vi "Downloader.vi"(4 "port":u16=9090, 6 "address":string="192.168.1.7", 7 "Message Box":refnum<vi>, 8 "error in":errorcluster, 11 "source":path=path "") -> (0 "error out":errorcluster, 3 "Downloader out":refnum<class "Downloader.lvclass">)   [LabVIEW 2014, in "Raspberry Pi Compatible Compiler for LabVIEW.lvlib" / "Downloader.lvclass"]
uses:
  Downloader.lvclass
  Downloader.lvclass/Downloader.ctl
  MessageBox/MessageBox.lvclass
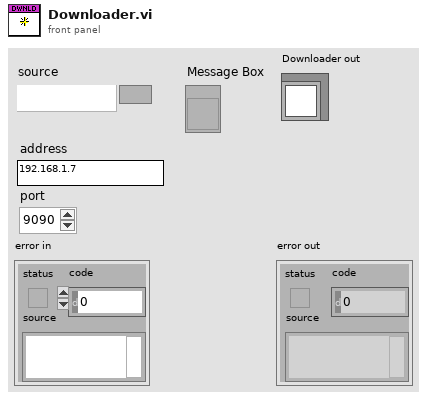
[diagram p1: front panel]
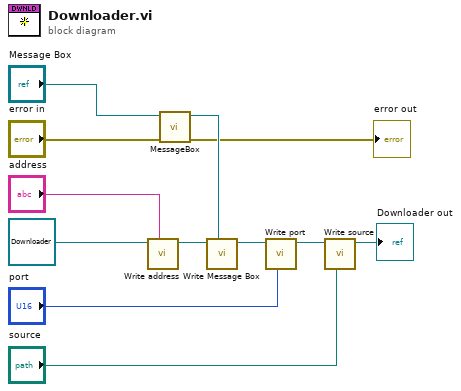
[diagram p0: block diagram]
diagram:
  n1 = call "Write address.vi"("address"="address", "Downloader in"=refnum<class "Downloader.lvclass"> refnum) -> ("Downloader out"=w12:refnum<class "Downloader.lvclass">)  [unwired: 7 in]
  n2 = call "MessageBox.vi"("error in"="error in", "Message Box"="Message Box") -> ("error out"=→"error out":errorcluster, "MessageBox out"=w3:refnum<class "MessageBox.lvclass">)  [unwired: 8 in]
  n3 = call "Write Message Box.vi"("Message Box"=w3, "Downloader in"=w12) -> ("Downloader out"=w11:refnum<class "Downloader.lvclass">)  [unwired: 7 in]
  n4 = call "Write port.vi"("port"="port", "Downloader in"=w11) -> ("Downloader out"=w10:refnum<class "Downloader.lvclass">)  [unwired: 7 in]
  n5 = call "Write source.vi"("source"="source", "Downloader in"=w10) -> ("Downloader out"=→"Downloader out":refnum<class "Downloader.lvclass">)  [unwired: 7 in]
